vi "02 RESTful API.vi"() -> ()   [LabVIEW 2019]
uses:
  _Subs/OpenDiagram/Open_XControl.xctl
  <vilib>/httpClient/LabVIEWHTTPClient.lvlib
panel:
  out "Property (str)":string
  in  "OpenDiag":refnum<vi>(xcontrol)
  # "02 RESTful API\nThis code goes online to get a Chuck Norris Joke \n\nInstructions:\n1. Connect your computer to the internet\n2. Hit Run and read the joke"
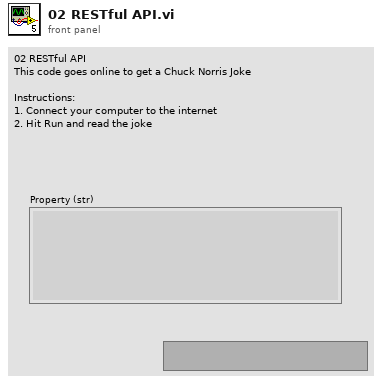
[diagram p1: front panel]
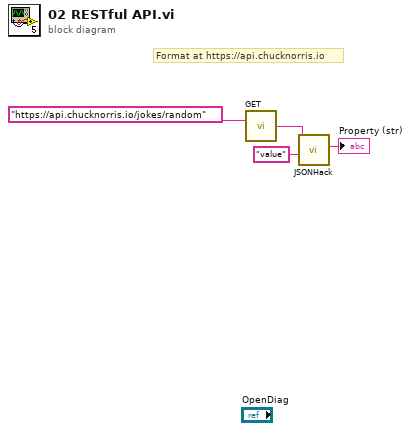
[diagram p0: block diagram]
diagram:
  # "Format at https://api.chucknorris.io"
  n1 = call <vilib>:"GET.vi"("url"="https://api.chucknorris.io/jokes/random") -> ("body"=w3:string)  [unwired: 11 in, 3 out]
  n2 = call "JSONHack.vi"("search name"="value", "JSON in"=w3) -> ("Property (str)"=→"Property (str)":string)  [unwired: 6 in, 3 out]
